vi "Download Stored Trip File.vi"(8 "error in (no error)":errorcluster, 10 "File Name":string, 11 "TCP Network Connection in":refnum<k5>) -> (0 "error out":errorcluster)   [LabVIEW 2020]
doc: "Author: Scott Hannahs <sth@magnet.fsu.edu>\nCopyright 2018 Florida State University, All rights reserved."
uses:
  TCP Functions/TCP Write Length and Data (U32).vi
  TCP Functions/TCP Write Length and Data (STR).vi
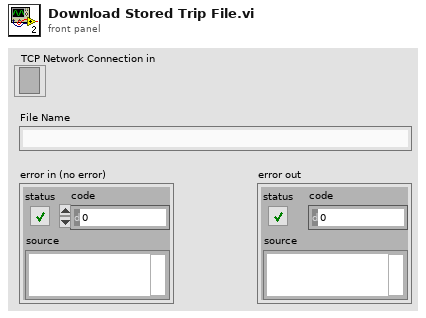
[diagram p1: front panel]
types:
  T1 = enum16{"open", "replace", "create", "open or create", "replace or create", "replace or create with confirmation"}
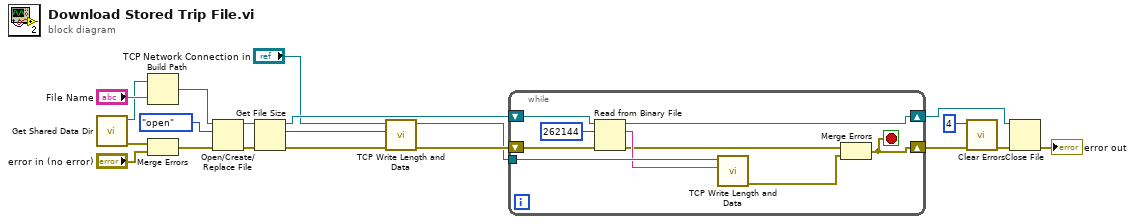
[diagram p0: block diagram]
diagram:
  n1 = call "Get Shared Data Dir.vi"() -> ("Error Out"=w1:errorcluster, "Data Directory Path"=w3:path)  [unwired: 2 in]
  n2 = Build Path(base path=w3, name or relative path="File Name") -> (appended path=w15:path)
  n3 = Merge Errors(w1, "error in (no error)") -> (w19:errorcluster)
  n4 = Open/Create/Replace File(file path (use dialog)=w15, error in=w19, operation (0:open)=T1."open") -> (refnum out=w20:refnum<file>, error out=w18:errorcluster)  [unwired: 3 in, 1 out]
  n5 = Get File Size(file=w20, error in=w18) -> (refnum out=w16:refnum<file>, size (in bytes)=w5:i64, 0:w10:errorcluster)
  n6 = call-poly "TCP Write Length and Data.vi"("Error In"=w10, "Data"=w5, "connection ID"="TCP Network Connection in") -> ("Error Out"=w17:errorcluster, "connection ID out"=w14:refnum<k5>)  [unwired: 7 in]
  n7 = while {
    shift-right: [w27] -> w9
    shift-left: w16 -> [w28]
    shift-right: [w22] -> w11
    shift-left: w17 -> [w26]
    tunnel: w14 -> [w25]
    stop <- w22 stop-if-true
    n8 = Read from Binary File(8:w26, 10:262144 ("count (1)"), 11:w28) -> (0:w21:errorcluster, 2:w24:string, 3:w27:refnum<file>)  [unwired: 3 in, 1 out]
    n9 = call-poly "TCP Write Length and Data.vi"("Data"=w24, "connection ID"=w25) -> ("Error Out"=w23:errorcluster)  [unwired: 8 in, 1 out]
    n10 = Merge Errors(w21, w23) -> (w22:errorcluster)
  }
  n11 = call <vilib>:"Clear Errors.vi"("error in (no error)"=w11, "specific error code to clear (0: all)"=4) -> ("error out"=w7:errorcluster)  [unwired: 4 in, 1 out]
  n12 = Close File(refnum=w9, error in=w7) -> (error out=→"error out":errorcluster)  [unwired: 1 out]
